vi "TrianglesScale.vi"(10 "ScaleFac":sgl, 11 "TrianglesIn":T1[](array[typedef])) -> (3 "TrianglesOut":T1[](array[typedef]))   [LabVIEW 2014]
uses:
  TypeDefs/TriangleFace.ctl
  TypeDefs/Point3D.ctl
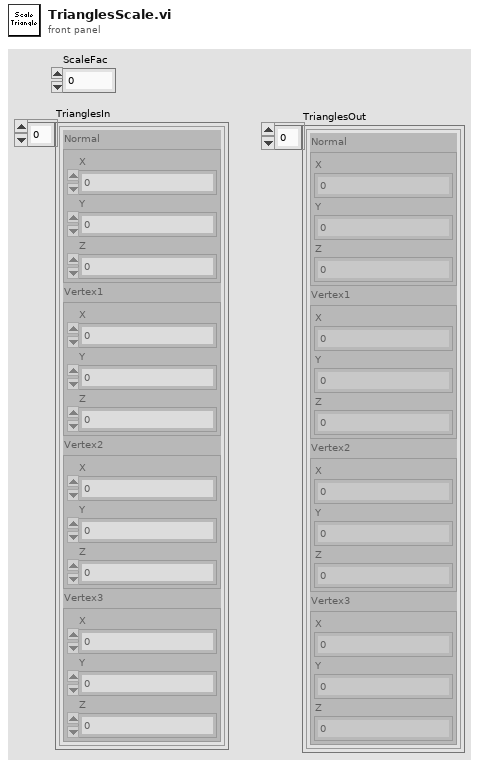
[diagram p1: front panel]
types:
  T1 = typedef "TriangleFace.ctl" = cluster{"Normal":T2, "Vertex1":T2, "Vertex2":T2, "Vertex3":T2}
  T2 = typedef "Point3D.ctl" = cluster{"X":sgl, "Y":sgl, "Z":sgl}
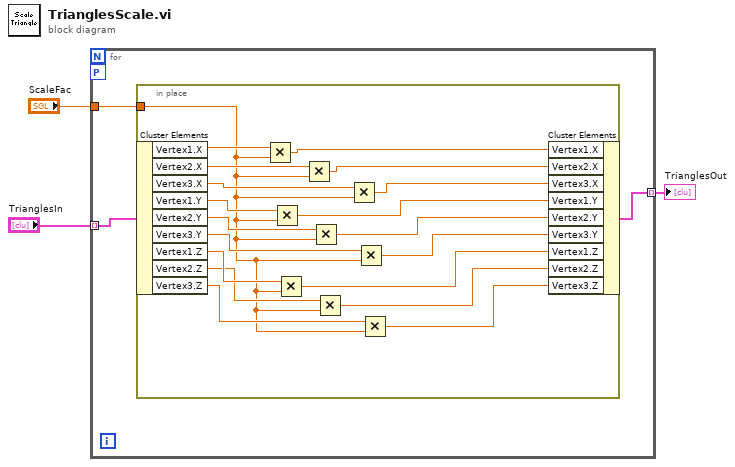
[diagram p0: block diagram]
diagram:
  n1 = for {
    tunnel: "TrianglesIn" -> [w6] mode=indexing
    tunnel: "ScaleFac" -> [w5]
    tunnel: [w4] -> w1 mode=indexing
    workers-P: _ -> [_]
    n2 = in-place {
      in-place-border: w5 -> [w10]
      n3 = in-place-cluster #1(w6) -> ("Vertex1.X"=w25:sgl, "Vertex2.X"=w24:sgl, "Vertex3.X"=w22:sgl, "Vertex1.Y"=w19:sgl, "Vertex2.Y"=w18:sgl, "Vertex3.Y"=w17:sgl, "Vertex1.Z"=w13:sgl, "Vertex2.Z"=w12:sgl, "Vertex3.Z"=w11:sgl)
      n4 = Multiply(x=w25, y=w10) -> (x*y=w20:sgl)
      n5 = Multiply(x=w19, y=w10) -> (x*y=w16:sgl)
      n6 = Multiply(x=w13, y=w10) -> (x*y=w9:sgl)
      n7 = Multiply(x=w24, y=w10) -> (x*y=w23:sgl)
      n8 = Multiply(x=w18, y=w10) -> (x*y=w15:sgl)
      n9 = Multiply(x=w12, y=w10) -> (x*y=w8:sgl)
      n10 = Multiply(x=w22, y=w10) -> (x*y=w21:sgl)
      n11 = Multiply(x=w17, y=w10) -> (x*y=w14:sgl)
      n12 = Multiply(x=w11, y=w10) -> (x*y=w7:sgl)
      n13 = in-place-cluster #1("Vertex1.X"=w20, "Vertex2.X"=w23, "Vertex3.X"=w21, "Vertex1.Y"=w16, "Vertex2.Y"=w15, "Vertex3.Y"=w14, "Vertex1.Z"=w9, "Vertex2.Z"=w8, "Vertex3.Z"=w7) -> (w4:T1)
    }
  }
  "TrianglesOut" <- w1
